vi "etlClose.vi"(1 "lens":enum16{"0", "1"}(ring)) -> ()   [LabVIEW 2017]
uses:
  globalDevices.vi
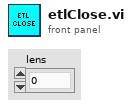
[diagram p1: front panel]
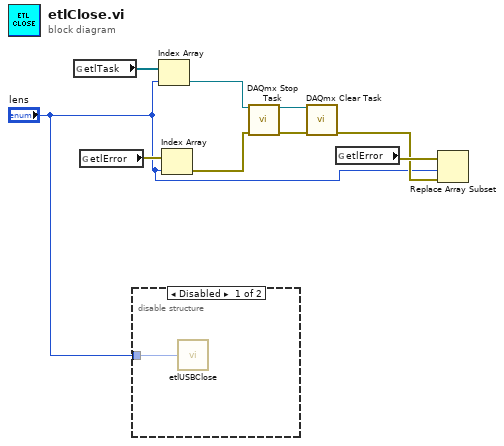
[diagram p0: block diagram]
diagram:
  n1 = global read "globalDevices.vi" "etlTask"() -> (w7:refnum<k21>[])
  n2 = global read "globalDevices.vi" "etlError"() -> (w6:errorcluster[])
  n3 = disable-structure shown="Disabled" {
    disable-tunnel: "lens" -> [w10 _]
    frame Disabled {
      n4 = call "etlUSBClose.vi"("lens"=w10) -> ()  [unwired: 1 in]
    }
    frame Enabled {
    }
  }
  n5 = Index Array(array=w7, index="lens") -> (element=w4:refnum<k21>)
  n6 = Index Array(array=w6, index="lens") -> (element=w5:errorcluster)
  n7 = call <vilib>:"DAQmx Stop Task.vi"("task/channels in"=w4, "error in"=w5) -> ("task out"=w9:refnum<k21>, "error out"=w8:errorcluster)  [unwired: 12 in]
  n8 = call <vilib>:"DAQmx Clear Task.vi"("task in"=w9, "error in"=w8) -> ("error out"=w2:errorcluster)  [unwired: 13 in]
  n9 = global read "globalDevices.vi" "etlError"() -> (w3:errorcluster[])
  n10 = Replace Array Subset(array=w3, new element=w2, index="lens") -> ()  [unwired: 1 out]
